vi "Email_Attachment_Plot.vi"(0 "controlRef":refnum<vi>, 1 "X axis name":string, 2 "Y axis name":string, 3 "XY Graph":cluster{dbl[], dbl[]}[](graph), 4 "Series Names":string[](array[string]), 5 "message":string, 6 "subject":string="[No Subject]") -> ()   [LabVIEW 2022 SP3]
uses:
  Email_transfer_global.vi
panel:
  in  "Tab Control":enum32{"Input", "Graph"}(tab)
  out "Plotted":string
  # "Either pass in a graph to be reproduced here, OR a reference to a control to be printed and attached to an email.\nPassing in a reference to a control allows ALL its formatting to be preserved"
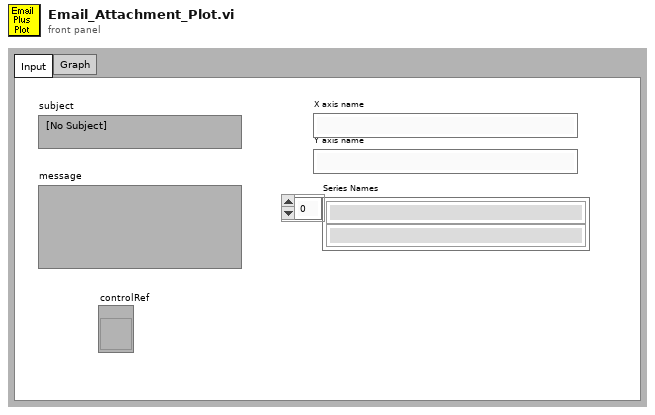
[diagram p1: front panel]
types:
  T1 = typedef "imagedata.ctl" = cluster{"image type":i32, "image depth":i32, "image":u8[], "mask":u8[], "colors":u32[], "Rectangle":cluster{"left":i16, "top":i16, "right":i16, "bottom":i16}}
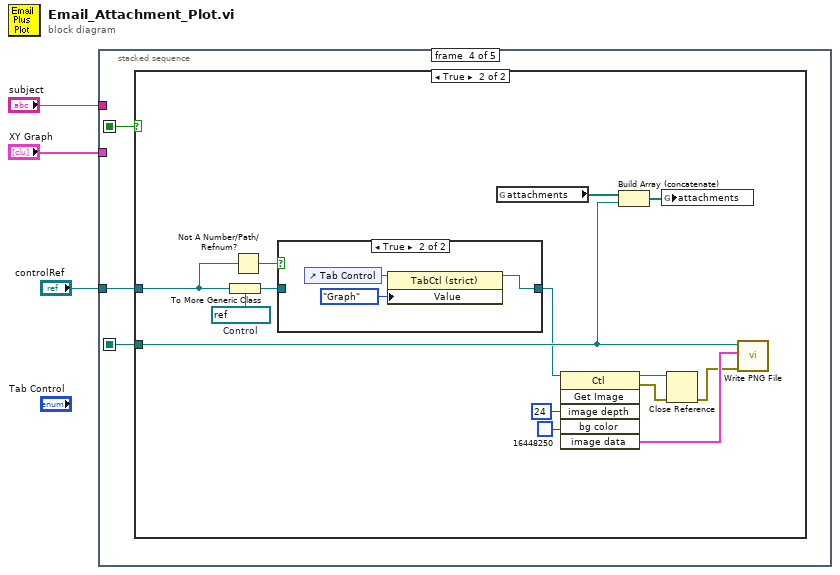
[diagram p0: block diagram]
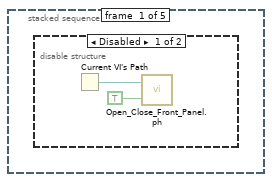
[diagram p2: hidden frame]
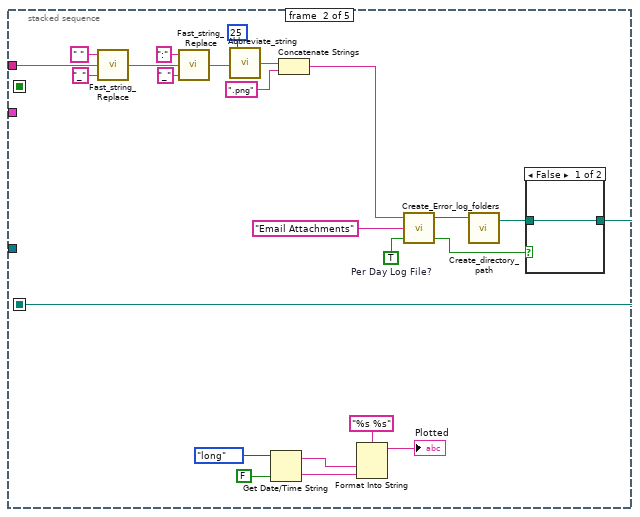
[diagram p4: hidden frame]
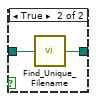
[diagram p5: hidden frame]
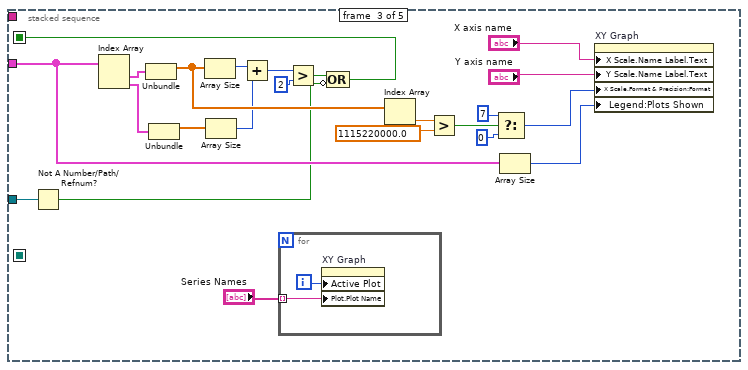
[diagram p6: hidden frame]
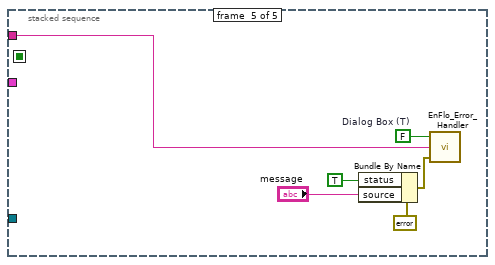
[diagram p9: hidden frame]
diagram:
  n1 = stacked-sequence {
    seq-local: [_ w9 _ _ _] -> [_ _ _ w59 _]
    seq-local: [_ _ w37 _ _] -> [_ _ _ w58 _]
    tunnel: "subject" -> [_ w17 _ _ w83]
    tunnel: "XY Graph" -> [_ _ w44 _ _]
    tunnel: "controlRef" -> [_ _ w38 w57 _]
    frame #0 {
      n2 = disable-structure shown="Disabled" {
        frame Disabled {
          n3 = Current VI's Path() -> (path=w4:path)
          n4 = call "Open_Close_Front_Panel.ph.vi"("openWindow (T)"=TRUE ("Front Panel Window:Open"), "VI path"=w4) -> ()  [unwired: 1 in, 1 out]
        }
        frame Enabled {
        }
      }
    }
    frame #1 {
      w6 = TRUE  # Per Day Log File?
      n5 = call "Fast_string_Replace.vi"("Replace match with:"="_", "Input String"=w17, "matchThis"=" " ("regular expression")) -> ("Output String"=w16:string)  [unwired: 1 in, 1 out]
      n6 = call "Fast_string_Replace.vi"("Replace match with:"="_", "Input String"=w16, "matchThis"=":" ("regular expression")) -> ("Output String"=w15:string)  [unwired: 1 in, 1 out]
      n7 = call "Abbreviate_string.vi"("Input String"=w15, "Max String Length"=25 ("length (rest)")) -> ("Output String"=w13:string)  [unwired: 1 in, 2 out]
      n8 = Get Date/Time String(date format (0)=enum16{"short", "long", "abbreviated"}."long", want seconds? (F)=FALSE) -> (date string=w25:string, time string=w24:string)  [unwired: 1 out]
      n9 = Concatenate Strings(w13, ".png" ("string")) -> (w11:string)
      n10 = Format Into String(format string="%s %s", w25, w24) -> (resulting string=→"Plotted":string)  [unwired: 2 in, 1 out]
      n11 = call "Create_Error_log_folders.vi"("Log Filename"=w11, "Log Folder"="Email Attachments" ("name or relative path"), "Per Day Log File?"=w6) -> ("Local Log File"=w8:path, "exists?"=w10:bool)  [unwired: 3 in]
      n12 = call "Create_directory_path.vi"("Path name"=w8) -> ("Path name Out"=w7:path)  [unwired: 2 in, 1 out]
      n13 = case shown="False" w10 {
        tunnel: w7 -> [w29 w31]
        tunnel: [w29 w30] -> w9
        frame False {
        }
        frame True {
          n14 = call "Find_Unique_Filename.vi"("Path In"=w31) -> ("Unique Path Out"=w30:path)  [unwired: 2 in]
        }
      }
    }
    frame #2 {
      n15 = Not A Number/Path/Refnum?(number/path/refnum=w38) -> (NaN/Path/Refnum?=w36:bool)
      n16 = Index Array(array=w44) -> (element #1=w46:cluster{dbl[], dbl[]}, element #2=w35:cluster{dbl[], dbl[]})  [unwired: 2 in]
      n17 = Unbundle(w46) -> (w40:dbl[])  [unwired: 1 out]
      n18 = Unbundle(w35) -> (w34:dbl[])  [unwired: 1 out]
      n19 = Array Size(array=w40) -> (size(s)=w41:i32)
      n20 = Array Size(array=w34) -> (size(s)=w32:i32)
      n21 = Add(x=w41, y=w32) -> (x+y=w33:i32)
      n22 = for {
        tunnel: "Series Names" -> [w55] mode=indexing
        i -> [w56]
        n23 = property on="XY Graph" class="XYGraph (strict)"("Active Plot"=w56, "Plot.Plot Name"=w55) -> ()  [unwired: 2 in, 2 out]
      }
      n24 = Greater?(x=w33, y=2) -> (0:w39:bool)
      n25 = Compound Arithmetic op=OR(w39, invert w36) -> (w37:bool)
      n26 = Index Array(array=w40) -> (element=w45:dbl)  [unwired: 1 in]
      n27 = Greater?(x=w45, y=1115220000.0) -> (0:w51:bool)
      n28 = Select(t=u8 7 ("Write Attribute"), s=w51, f=u8 0 ("Write Attribute")) -> (s? t:f=w47:u8)
      n29 = Array Size(array=w44) -> (size(s)=w43:i32)
      n30 = property on="XY Graph" class="XYGraph (strict)"("X Scale.Name Label.Text"="X axis name", "Y Scale.Name Label.Text"="Y axis name", "X Scale.Format & Precision:Format"=w47, "Legend:Plots Shown"=w43) -> ()  [unwired: 2 in, 2 out]
    }
    frame #3 {
      n31 = case shown="True" w58 {
        tunnel: w59 -> [_ w71]
        tunnel: w57 -> [_ w60]
        frame False {
          # "Nothing to plot"
        }
        frame True {
          w69 = refnum<vi> refnum  # Control
          n32 = To More Generic Class(target class=w69, reference=w60) -> (generic class reference=w63:refnum<vi>)
          n33 = Not A Number/Path/Refnum?(number/path/refnum=w60) -> (NaN/Path/Refnum?=w65:bool)
          n34 = case shown="True" w65 {
            tunnel: [w74 w75] -> w64
            tunnel: w63 -> [w74 _]
            frame False {
            }
            frame True {
              n35 = control-ref of="Tab Control"() -> (w77:refnum<vi>)
              n36 = property class="TabCtl (strict)"(reference=w77, "Value"=enum32{"Input", "Graph"}."Graph") -> (reference out=w75:refnum<vi>)  [unwired: 1 in, 1 out]
            }
          }
          n37 = global read "Email_transfer_global.vi" "attachments"() -> (w73:path[])
          n38 = invoke class="Ctl" method="Get Image"(reference=w64, "image depth"=24 ("Image Depth"), "bg color"=u32 16448250 ("Background Color")) -> (reference out=w68:refnum<vi>, error out=w67:errorcluster, "image data"=w70:T1)  [unwired: 3 in, 3 out]
          n39 = Build Array (concatenate)(w73, w71) -> (w72:path[])
          n40 = global write "Email_transfer_global.vi" "attachments"(w72) -> ()
          n41 = Close Reference(reference=w68, error in (no error)=w67) -> (error out=w66:errorcluster)
          n42 = call <vilib>:"Write PNG File.vi"("error in (no error)"=w66, "image data"=w70, "path to PNG file"=w71) -> ()  [unwired: 7 in, 2 out]
        }
      }
    }
    frame #4 {
      w78 = FALSE  # Dialog Box (T)
      n43 = Bundle By Name(cluster=errorcluster {"status"=FALSE, "code"=0, "source"=""} ("error in (no error)"), "status"=TRUE, "source"="message") -> (w81:errorcluster)
      n44 = call "EnFlo_Error_Handler.vi"("error in (no error)"=w81, "Error Type"=w83, "Dialog Box (F)"=w78) -> ()  [unwired: 3 out]
    }
  }
